vi "ProjectSearchDataName.vi"(8 "error in (no error)":errorcluster, 11 "element":string) -> (0 "error out":errorcluster, 1 "Index":cluster{"Y":i32, "X":i32}, 2 "variant":variant, 3 "DataOut":string)   [LabVIEW 2019]
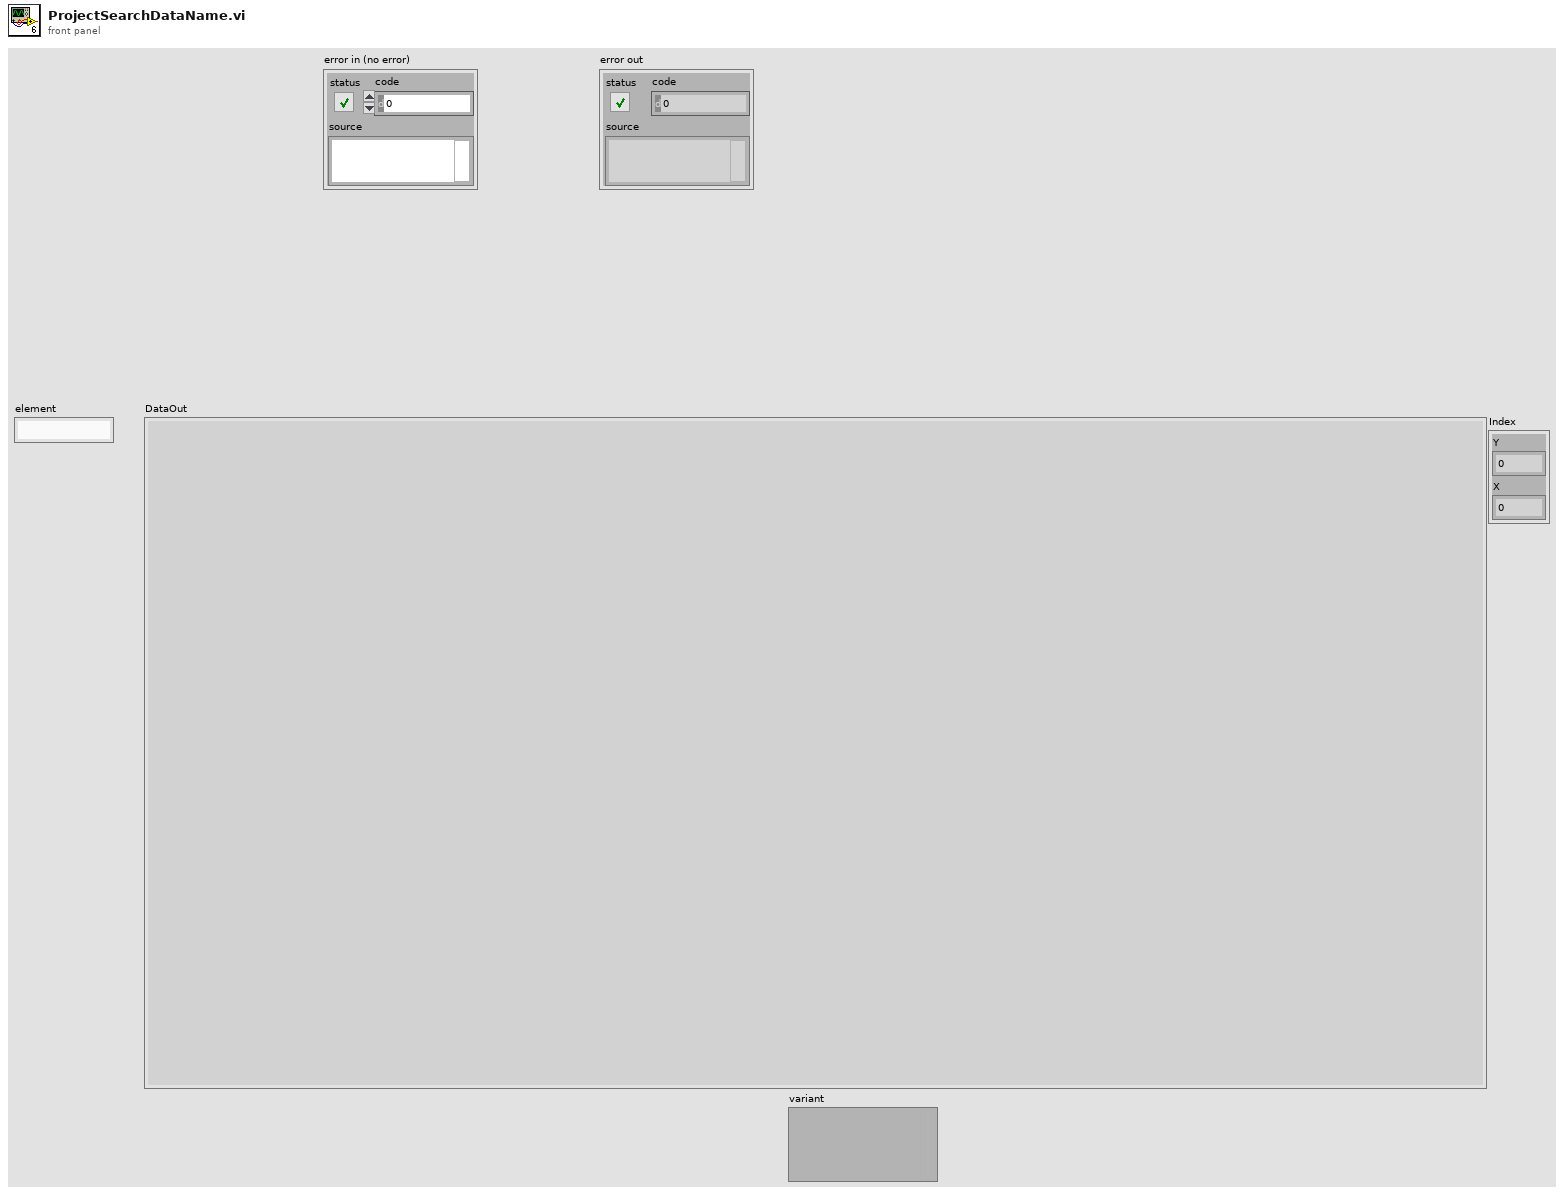
[diagram p1: front panel]
types:
  T1 = cluster{"type string":i16[], "data string":string}
  T2 = enum16{"initial", "save", "load", "write", "read"}
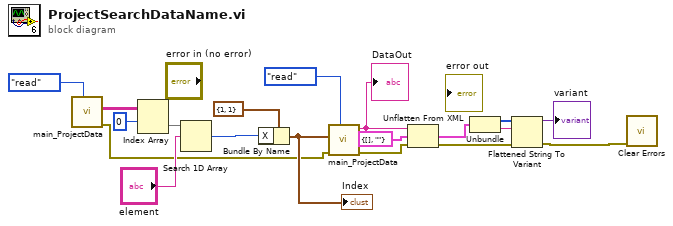
[diagram p0: block diagram]
diagram:
  n1 = call "main_ProjectData.vi"("Enum"=T2."read") -> ("error out"=w2:errorcluster, "Table Control"=w12:string[][])  [unwired: 8 in, 1 out]
  n2 = Index Array(array=w12, index (row)=0) -> (element=w14:string[])  [unwired: 1 in]
  n3 = Search 1D Array(1D array=w14, element="element") -> (index of element=w18:i32)  [unwired: 1 in]
  n4 = Bundle By Name(cluster=cluster{"Y":i32, "X":i32} {"Y"=1, "X"=1} ("Index"), "X"=w18) -> (w19:cluster{"Y":i32, "X":i32})
  "Index" <- w19
  n5 = call "main_ProjectData.vi"("Enum"=T2."read", "error in"=w2, "Index"=w19) -> ("error out"=w1:errorcluster, "DataOut"=w5:string)  [unwired: 6 in, 1 out]
  "DataOut" <- w5
  n6 = Unflatten From XML(xml string=w5, type=T1 {"type string"=[], "data string"=""} ("cluster"), error in (no error)=w1) -> (value=w9:T1, error out=w6:errorcluster)
  n7 = Unbundle(w9) -> ("type string"=w8:i16[], "data string"=w7:string)
  n8 = Flattened String To Variant(4:w6, 6:w7, 7:w8) -> (0:w3:errorcluster, 3:→"variant":variant)
  n9 = call <vilib>:"Clear Errors.vi"("error in (no error)"=w3) -> ()  [unwired: 5 in, 2 out]
